vi "SD1 Test.vi"() -> ()   [LabVIEW 2019]
panel:
  out "errorOut":errorcluster
  in  "partNumber":string
  in  "nChassis":i32
  in  "nSlot":i32
  in  "errorIn":errorcluster
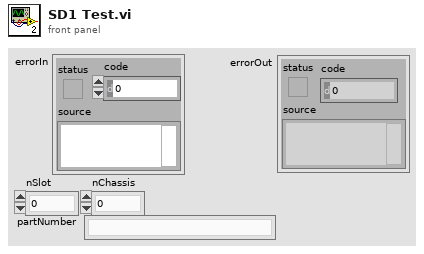
[diagram p1: front panel]
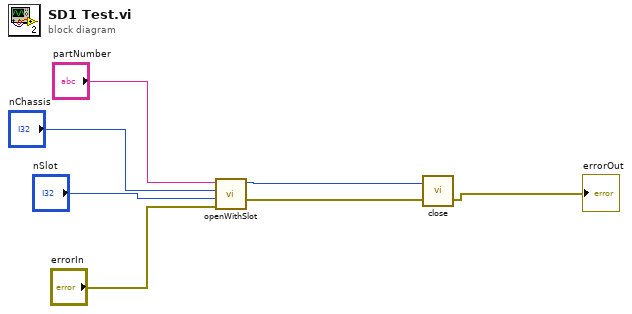
[diagram p0: block diagram]
diagram:
  n1 = call <vilib>:"openWithSlot.vi"("errorIn"="errorIn", "nSlot"="nSlot", "nChassis"="nChassis", "partNumber"="partNumber") -> ("errorOut"=w2:errorcluster, "moduleID"=w1:i32)  [unwired: 2 in]
  n2 = call <vilib>:"close.vi"("errorIn"=w2, "moduleID"=w1) -> ("errorOut"=→"errorOut":errorcluster)  [unwired: 1 in]
